vi "relay_action(moose).vi"(0 "VISA resource name":refnum<visa-resource-name>="ASRL2::INSTR", 1 "init?":bool=TRUE, 2 "Port Configuration":T1={"baud rate (9600)"=9600, "data bits (8)"=8, "parity (0:none)"=enum."None", "stop bits (10: 1 bit)"=10, "flow control (0:none)"=0, "timeout (10sec)"=10000, "termination char\n(0xA = '\\n' = LF) "=10, "Enable Termination\nChar (T)"=TRUE} {"termination char\n(0xA = '\\n' = LF)" format="%.0x"; "flow control (0:none)" items=["None", "XON/XOFF", "RTS/CTS", "XON/XOFF & RTS/CTS", "DTR/DSR", "XON/XOFF & DTR/DSR"]; "stop bits (10: 1 bit)" items=["1.0"=10, "1.5"=15, "2.0"=20]; "data bits (8)" min=5 max=8 step=1}, 3 "Action":u8(ring) items=["open dump on"=8, "pump acid on"=9, "air flush on"=10, "stop gas flow on"=11, "open dump off"=0, "pump acid off"=1, "air flush on"=2, "stop gas flow on"=3, "OpenAll"=30, "CloseAll"=29], 4 "Quit?":bool=TRUE, 5 "error in":errorcluster) -> (6 "VISA resource name 2":refnum<visa-resource-name>="ASRL2::INSTR", 8 "error out":errorcluster)   [LabVIEW 2010]
uses:
  <vilib>/Instr/_visa.llb/VISA Configure Serial Port (Instr).vi
panel:
  out "code":u8=254
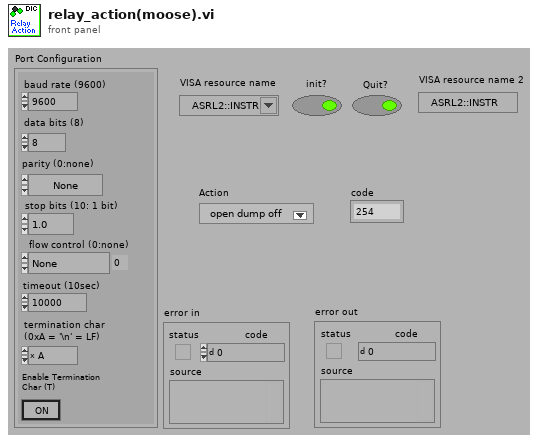
[diagram p1: front panel]
types:
  T1 = cluster{"baud rate (9600)":u32, "data bits (8)":u16, "parity (0:none)":enum16{"None", "Odd", "Even", "Mark", "Space"}, "stop bits (10: 1 bit)":u16, "flow control (0:none)":u16, "timeout (10sec)":u32, "termination char\n(0xA = '\\n' = LF) ":u8, "Enable Termination\nChar (T)":bool}
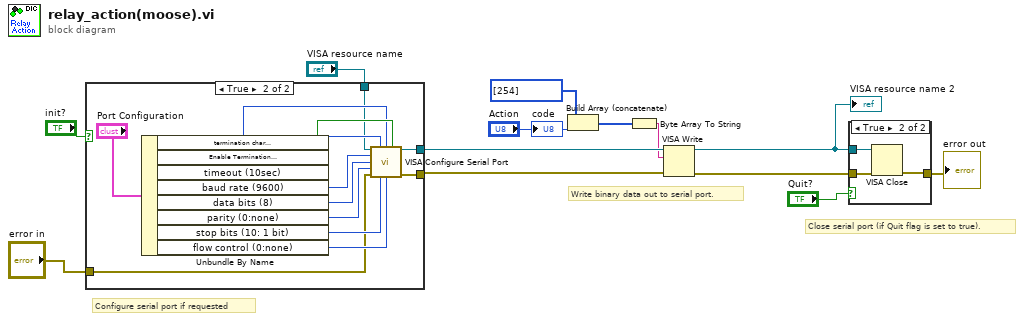
[diagram p0: block diagram]
diagram:
  # "Close serial port (if Quit flag is set to true)."
  # "Write binary data out to serial port."
  # "Configure serial port if requested"
  n1 = case shown="True" "init?" {
    tunnel: [w14 w19] -> w11
    tunnel: [w15 w18] -> w10
    tunnel: "error in" -> [w15 w17]
    tunnel: "VISA resource name" -> [w14 w16]
    frame False {
    }
    frame True {
      n2 = Unbundle By Name("Port Configuration") -> ("termination char\n(0xA = '\\n' = LF)"=w20:u8, "Enable Termination\nChar (T)"=w21:bool, "timeout (10sec)"=w22:u32, "baud rate (9600)"=w27:u32, "data bits (8)"=w26:u16, "parity (0:none)"=w25:enum16{"None", "Odd", "Even", "Mark", "Space"}, "stop bits (10: 1 bit)"=w24:u16, "flow control (0:none)"=w23:u16)
      n3 = call-poly "VISA Configure Serial Port"("VISA resource name"=w16, "timeout (10sec)"=w22, "termination char\n(0xA = '\\n' = LF)"=w20, "Enable Termination\nChar (T)"=w21, "baud rate (9600)"=w27, "data bits (8)"=w26, "parity (0:none)"=w25, "error in (no error)"=w17, "stop bits (10: 1 bit)"=w24, "flow control (0:none)"=w23) -> ("VISA resource name out"=w19:refnum<visa-resource-name>, "error out"=w18:errorcluster)  [unwired: 4 in]
    }
  }
  n4 = Build Array (concatenate)(u8[] [254] ("unsigned byte array"), "Action") -> (w5:u8[])
  n5 = Byte Array To String(unsigned byte array=w5) -> (string=w7:string)
  n6 = VISA Write(VISA resource name=w11, write buffer=w7, error in (no error)=w10) -> (VISA resource name out=w1:refnum<visa-resource-name>, error out=w13:errorcluster)  [unwired: 1 out]
  "VISA resource name 2" <- w1
  n7 = case shown="True" "Quit?" {
    tunnel: w1 -> [_ w30]
    tunnel: w13 -> [w29 w32]
    tunnel: [w29 w31] -> w3
    frame False {
    }
    frame True {
      n8 = VISA Close(VISA resource name=w30, error in (no error)=w32) -> (error out=w31:errorcluster)
    }
  }
  "error out" <- w3
  "code" <- "Action"
